vi "Configure FFT.vi"(7 "Enable FFT Display (T: Enable)":bool=TRUE, 8 "error in (no error)":errorcluster, 9 "FFT Window (0: Hanning)":i32(ring) items=["Hanning", "Flattop", "Rectangular"], 10 "FFT Channel (0: Channel 1)":i32(ring) items=["Channel 1", "Channel 2"], 11 "VISA resource name":refnum<visa-resource-name>) -> (0 "error out":errorcluster, 3 "VISA resource name out":refnum<visa-resource-name>)   [LabVIEW 2012, in "Tektronix TDS 200 1000 2000 Series.lvlib"]
doc: "Configures FFT and associated parameters.\n\n<B>Note(s):</b>\nAvailable on TBS1000B-EDU and TBS1000B series only."
uses:
  <instrlib>/Tektronix TDS 200 1000 2000 Series/Tektronix TDS 200 1000 2000 Series.lvlib
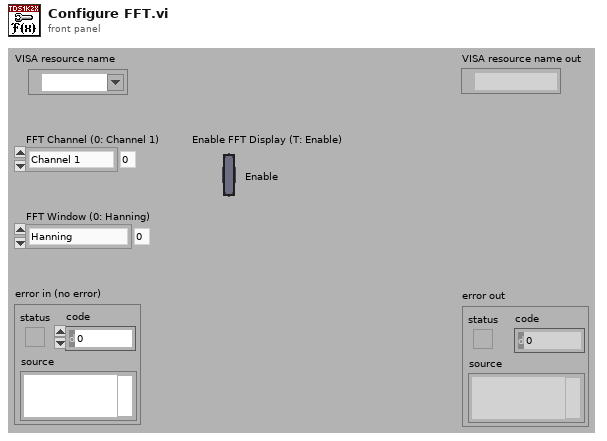
[diagram p1: front panel]
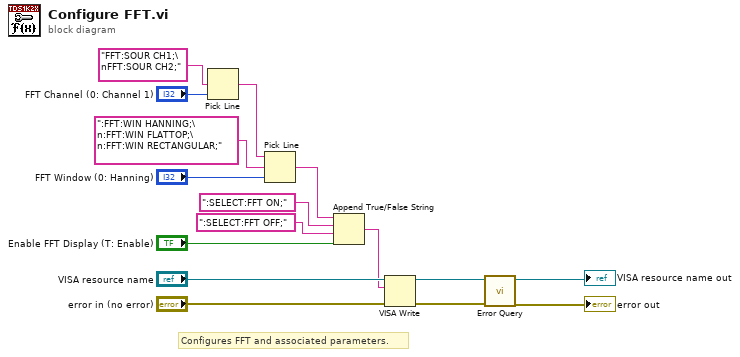
[diagram p0: block diagram]
diagram:
  # "Configures FFT and associated parameters."
  n1 = Pick Line(multi-line string="FFT:SOUR CH1;\nFFT:SOUR CH2;", line index="FFT Channel (0: Channel 1)") -> (output string=w12:string)  [unwired: 1 out]
  n2 = Pick Line(string ("")=w12, multi-line string=":FFT:WIN HANNING;\n:FFT:WIN FLATTOP;\n:FFT:WIN RECTANGULAR;", line index="FFT Window (0: Hanning)") -> (output string=w11:string)
  n3 = Append True/False String(1:"Enable FFT Display (T: Enable)", 2:":SELECT:FFT OFF;", 3:":SELECT:FFT ON;", 4:w11) -> (0:w2:string)
  n4 = VISA Write(VISA resource name="VISA resource name", write buffer=w2, error in (no error)="error in (no error)") -> (VISA resource name out=w6:refnum<visa-resource-name>, error out=w5:errorcluster)  [unwired: 1 out]
  n5 = call <instrlib>:"Error Query.vi"("error in (no error)"=w5, "VISA resource name"=w6) -> ("error out"=→"error out":errorcluster, "VISA resource name out"=→"VISA resource name out":refnum<visa-resource-name>)  [unwired: 8 out]
